vi "Get Turbo Valve Value.vi"(8 "error in (no error)":errorcluster, 11 "ILC Closed Loop Actuator Cylinder in":refnum<class "ILC Closed Loop Actuator Cylinder.lvclass">) -> (0 "error out":errorcluster, 2 "Value":dbl format="%.2f", 3 "ILC Closed Loop Actuator Cylinder out":refnum<class "ILC Closed Loop Actuator Cylinder.lvclass">)   [LabVIEW 2015, in "ILC Closed Loop Actuator Cylinder.lvclass"]
uses:
  ILC Closed Loop Actuator Cylinder.lvclass
  ILC Actuator Cylinder/ILC Actuator Cylinder.lvclass/ILC Actuator Cylinder.ctl
  ILC Closed Loop Actuator Cylinder.lvclass/ILC Closed Loop Actuator Cylinder.ctl
  <vilib>/addons/control/pid/pid.llb/PID (DBL).vi
  <vilib>/addons/control/pid/NI_PID_pid.lvlib
  ILC Actuator Cylinder/ILC Actuator Cylinder.lvclass
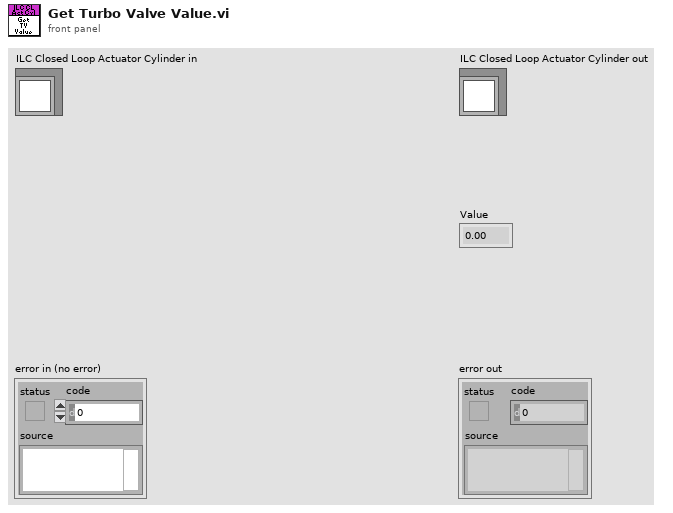
[diagram p1: front panel]
types:
  T1 = cluster{"proportional gain (Kc)":dbl, "integral time (Ti, min)":dbl, "derivative time (Td, min)":dbl}
  T2 = typedef "FAMT Typedefs.lvlib/PID Settings.ctl" = cluster{"Pressure Servo Valve Settings":T3, "Turbo Valve Settings":T3}
  T3 = typedef "FAMT Typedefs.lvlib/Closed Loop Settings.ctl" = cluster{"P":dbl, "I":dbl, "D":dbl, "Minimum":dbl, "Maximum":dbl}
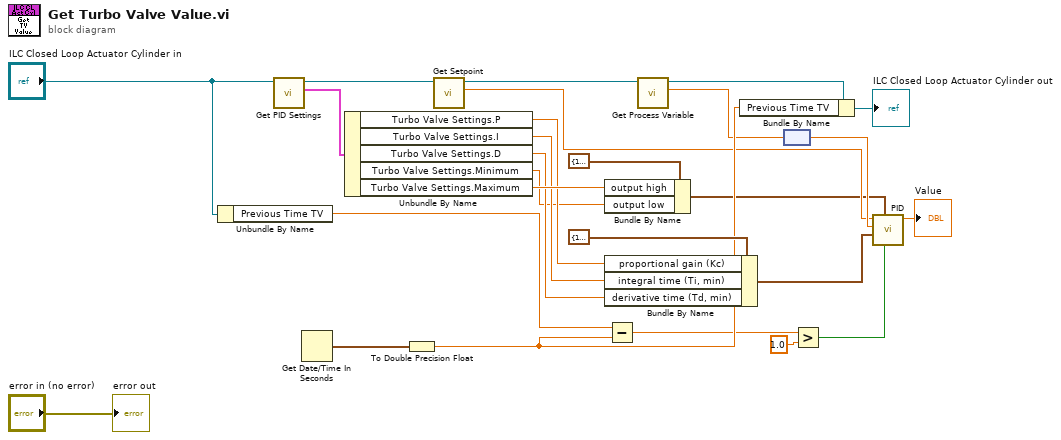
[diagram p0: block diagram]
diagram:
  n1 = Unbundle By Name("ILC Closed Loop Actuator Cylinder in") -> ("Previous Time TV"=w12:dbl)
  n2 = call "Get PID Settings.vi"("ILC Actuator Cylinder in"="ILC Closed Loop Actuator Cylinder in") -> ("PID Settings"=w13:T2, "ILC Actuator Cylinder out"=w11:refnum<class "ILC Closed Loop Actuator Cylinder.lvclass">)  [unwired: 9 in]
  n3 = Get Date/Time In Seconds() -> (seconds since 1Jan1904=w17:timestamp)
  n4 = Unbundle By Name(w13) -> ("Turbo Valve Settings.P"=w21:dbl, "Turbo Valve Settings.I"=w20:dbl, "Turbo Valve Settings.D"=w19:dbl, "Turbo Valve Settings.Minimum"=w18:dbl, "Turbo Valve Settings.Maximum"=w23:dbl)
  n5 = To Double Precision Float(number=w17) -> (double precision float=w16:dbl)
  n6 = call-dynamic "Get Setpoint.vi"("ILC Actuator Cylinder in"=w11) -> ("Setpoint"=w4:dbl, "ILC Actuator Cylinder out"=w10:refnum<class "ILC Closed Loop Actuator Cylinder.lvclass">)  [unwired: 9 in]
  n7 = Bundle By Name(cluster=cluster{"output high":dbl, "output low":dbl} {"output high"=100.0, "output low"=-100.0} ("output range"), "output high"=w23, "output low"=w18) -> (w3:cluster{"output high":dbl, "output low":dbl})
  n8 = Bundle By Name(cluster=T1 {"proportional gain (Kc)"=1.0, "integral time (Ti, min)"=0.01, "derivative time (Td, min)"=0.0} ("PID gains"), "proportional gain (Kc)"=w21, "integral time (Ti, min)"=w20, "derivative time (Td, min)"=w19) -> (w2:T1)
  n9 = Subtract(x=w12, y=w16) -> (x-y=w15:dbl)
  n10 = call-dynamic "Get Process Variable.vi"("ILC Actuator Cylinder in"=w10) -> ("Process Variable"=w8:dbl[unit], "ILC Actuator Cylinder out"=w9:refnum<class "ILC Closed Loop Actuator Cylinder.lvclass">)  [unwired: 9 in]
  n11 = Bundle By Name(cluster=w9, "Previous Time TV"=w16) -> (→"ILC Closed Loop Actuator Cylinder out":refnum<class "ILC Closed Loop Actuator Cylinder.lvclass">)
  n12 = node(w8) -> (w5:dbl)
  n13 = Greater?(x=w15, y=1.0) -> (0:w1:bool)
  n14 = call-poly <vilib>:"PID.vi"("reinitialize? (F)"=w1, "output range"=w3, "PID gains"=w2, "process variable"=w5, "setpoint"=w4) -> ("output"=→"Value":dbl)  [unwired: 5 in, 1 out]
  "error out" <- "error in (no error)"
